vi "Get_DXF.vi"(7 "Save as":string="PartStudio1", 8 "error in":errorcluster, 9 "Part Id":string="JMe", 10 "microversion":string="697dc900779ec9c32628a06b", 11 "Device In":T1) -> (0 "error out":errorcluster, 2 "Comm":T2, 3 "Device Out":T1, 4 "DXF Text":string)   [LabVIEW 2019]
uses:
  <userlib>/Onshape/_SubVI/Cluster.ctl
  <userlib>/IoT Devices/_subVIs/HTTPComm.ctl
  <userlib>/Onshape/_SubVI/z did wid and eid.vi
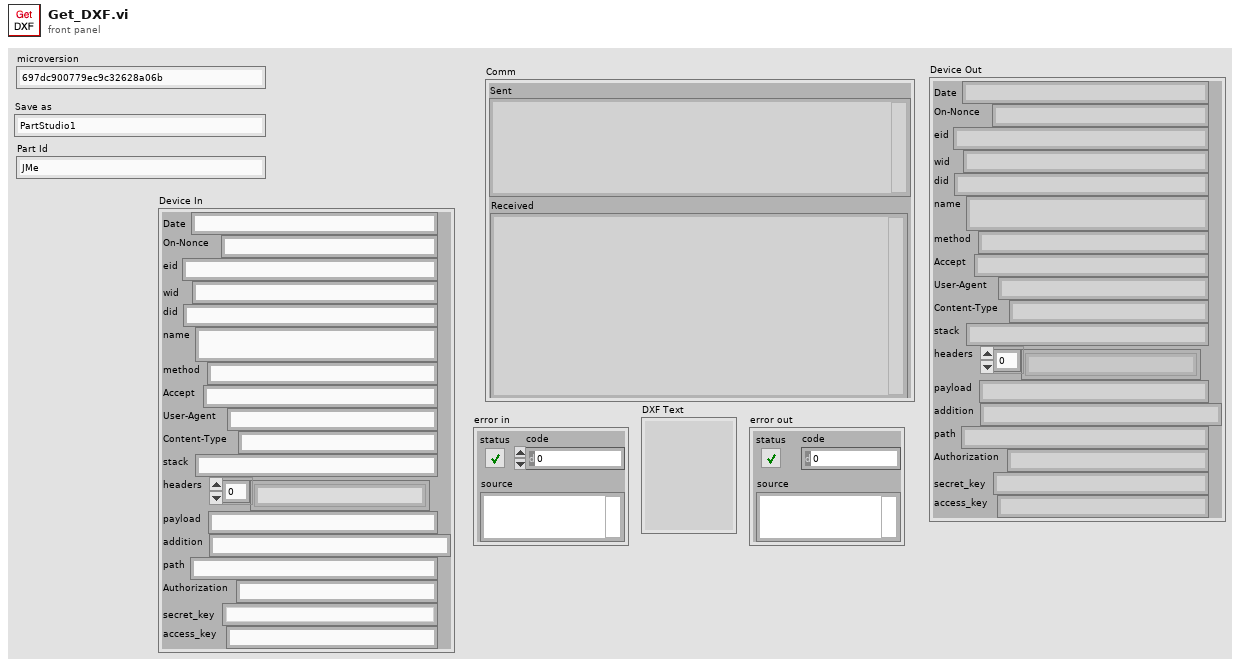
[diagram p1: front panel]
types:
  T1 = typedef "Cluster.ctl" = cluster{"Date":string, "On-Nonce":string, "eid":string, "wid":string, "did":string, "name":string, "method":string, "Accept":string, "User-Agent":string, "Content-Type":string, "stack":string, "headers":string[], "payload":string, "addition":string, "path":string, "Authorization":string, "secret_key":string, "access_key":string}
  T2 = typedef "HTTPComm.ctl" = cluster{"url":string, "sent headers":string, "sent body":string, "headers":string, "body":string, "Sent":string, "Received":string}
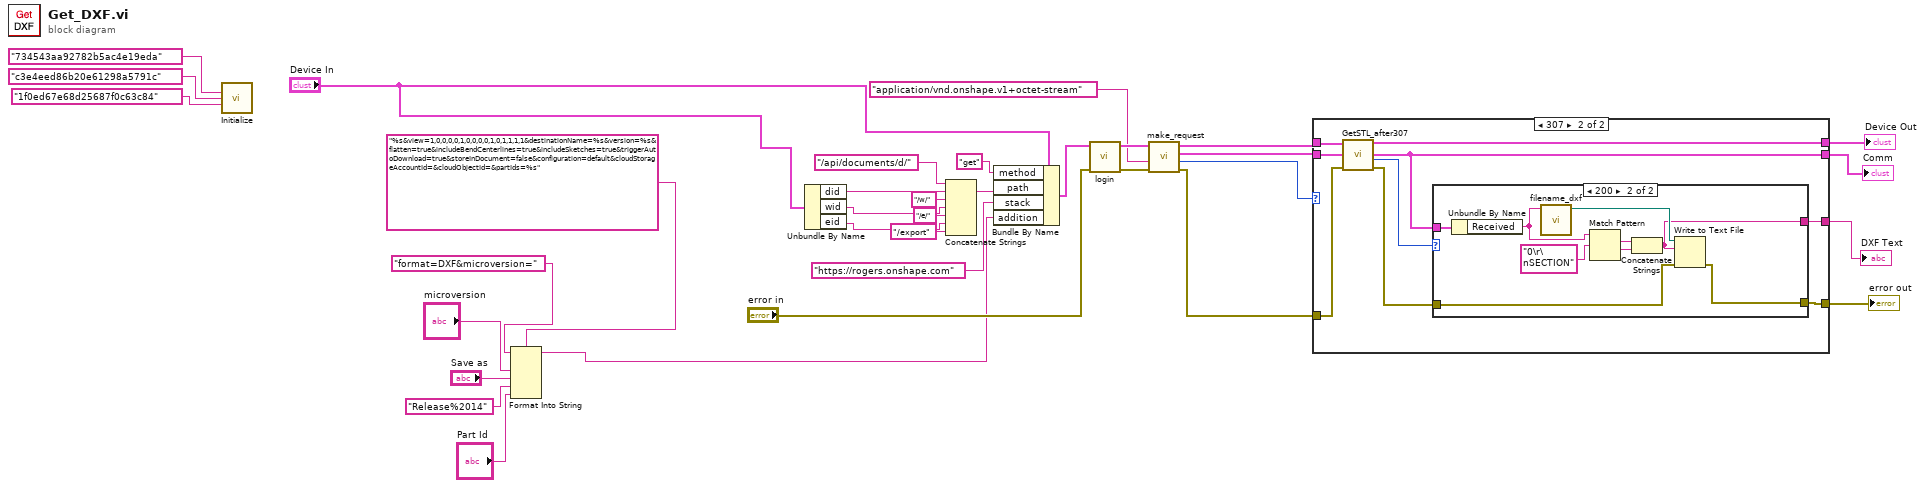
[diagram p0: block diagram]
diagram:
  n1 = call-poly <userlib>:"Initialize.vi"("did"="734543aa92782b5ac4e19eda", "wid"="c3e4eed86b20e61298a5791c", "eid"="1f0ed67e68d25687f0c63c84") -> ()  [unwired: 11 in, 2 out]
  n2 = Format Into String(format string="%s&view=1,0,0,0,0,1,0,0,0,0,1,0,1,1,1,1&destinationName=%s&version=%s&flatten=true&includeBendCenterlines=true&includeSketches=true&triggerAutoDownload=true&storeInDocument=false&configuration=default&cloudStorageAccountId=&cloudObjectId=&partIds=%s", initial string="format=DXF&microversion=", "microversion", "Save as", "Release%2014" ("input 3"), "Part Id") -> (resulting string=w8:string)  [unwired: 1 in, 1 out]
  n3 = Unbundle By Name("Device In") -> ("did"=w27:string, "wid"=w23:string, "eid"=w21:string)
  n4 = Concatenate Strings("/api/documents/d/" ("payload"), w27, "/w/" ("string"), w23, "/e/" ("string"), w21, "/export" ("string")) -> (w32:string)
  n5 = Bundle By Name(cluster="Device In", "method"="get" ("Method"), "path"=w32, "stack"="https://rogers.onshape.com" ("stacks"), "addition"=w8) -> (w29:T1)
  n6 = call <userlib>:"login.vi"("error in"="error in", "Device In"=w29) -> ("error out"=w30:errorcluster, "Device Out"=w28:T1)  [unwired: 8 in]
  n7 = call <userlib>:"make_request.vi"("Error in"=w30, "Accept"="application/vnd.onshape.v1+octet-stream", "Device In"=w28) -> ("error out"=w18:errorcluster, "error"=w19:i32, "Comm"=w17:T2, "Device Out"=w16:T1)  [unwired: 4 in, 1 out]
  n8 = case shown="307" w19 {
    tunnel: w18 -> [w35 w46]
    tunnel: w17 -> [w36 w45]
    tunnel: w16 -> [w37 w44]
    tunnel: [w37 w43] -> w15
    tunnel: [w36 w42] -> w14
    tunnel: [w35 w39] -> w13
    tunnel: [_ w38] -> w12
    frame 0, Default {
    }
    frame 307 {
      n9 = call <userlib>:"GetSTL_after307.vi"("error in (no error)"=w46, "Comm in"=w45, "Device in"=w44) -> ("error out"=w40:errorcluster, "error"=w41:i32, "Comm out"=w42:T2, "Device Out"=w43:T1)  [unwired: 5 in]
      n10 = case shown="200" w41 {
        tunnel: w42 -> [_ w56]
        tunnel: [w47 w49] -> w39
        tunnel: w40 -> [w47 w50]
        tunnel: [_ w48] -> w38
        frame 0, Default {
        }
        frame 200 {
          n11 = Unbundle By Name(w56) -> ("Received"=w52:string)
          n12 = call "filename_dxf.vi"("Received"=w52) -> ("appended path"=w51:path)  [unwired: 10 in]
          n13 = Match Pattern(string=w52, regular expression="0\r\nSECTION") -> (match substring=w54:string, after substring=w53:string)  [unwired: 1 in, 2 out]
          n14 = Concatenate Strings(w54, w53) -> (w48:string)
          n15 = Write to Text File(file (use dialog)=w51, text=w48, error in=w50) -> (error out=w49:errorcluster)  [unwired: 1 in, 2 out]
        }
      }
    }
  }
  "Device Out" <- w15
  "Comm" <- w14
  "error out" <- w13
  "DXF Text" <- w12
